vi "Map to Feet.vi"(9 "Draw Area Size":T1, 10 "Position":T2, 11 "Coords (px)":T3) -> (3 "Point (ft)":cluster{dbl, dbl})   [LabVIEW 2019]
uses:
  <vilib>/Utility/miscctls.llb/LVPoint32TypeDef.ctl
  <vilib>/Utility/miscctls.llb/LVPositionTypeDef.ctl
  <vilib>/Utility/miscctls.llb/LVBoundsTypeDef.ctl
  Globals.vi
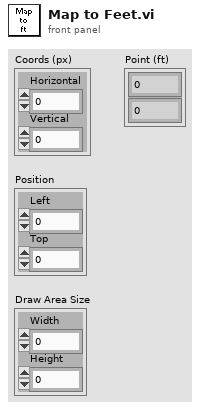
[diagram p1: front panel]
types:
  T1 = typedef "LVBoundsTypeDef.ctl" = cluster{"Width":u32, "Height":u32}
  T2 = typedef "LVPositionTypeDef.ctl" = cluster{"Left":i32, "Top":i32}
  T3 = typedef "LVPoint32TypeDef.ctl" = cluster{"Horizontal":i32, "Vertical":i32}
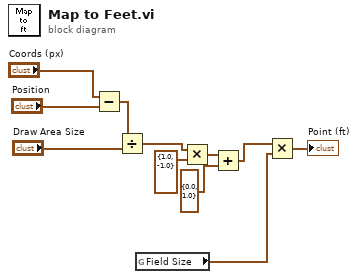
[diagram p0: block diagram]
diagram:
  n1 = Subtract(x="Coords (px)", y="Position") -> (x-y=w6:T3)
  n2 = Divide(x=w6, y="Draw Area Size") -> (x/y=w10:cluster{dbl, dbl})
  n3 = global read "Globals.vi" "Field Size"() -> (w1:cluster{"width":dbl, "height":dbl})
  n4 = Multiply(x=w10, y=cluster{"Width":dbl, "Height":dbl} {"Width"=1.0, "Height"=-1.0} ("Bounds")) -> (x*y=w8:cluster{dbl, dbl})
  n5 = Add(x=w8, y=cluster{"Width":dbl, "Height":dbl} {"Width"=0.0, "Height"=1.0} ("Bounds")) -> (x+y=w11:cluster{dbl, dbl})
  n6 = Multiply(x=w11, y=w1) -> (x*y=→"Point (ft)":cluster{dbl, dbl})
